vi "NEW Set Controller Limits.vi"(0 "IndMin":dbl, 1 "Min":dbl, 2 "Max":dbl, 3 "StepSize":dbl, 7 "ControlArray In":T1(array[cluster])=[{"Name"="Volt_Direct", "PI Far->Close"=[{"Slew"=1000.0, "Kp"=0.1, "Ki"=0.02}, {"Slew"=60.0, "Kp"=5.0, "Ki"=2.0}, {"Slew"=1.0, "Kp"=180.0, "Ki"=0.0}], "Limits"={"StepSize"=1e-05, "Max"=10.0, "Min"=0.0, "IndMin"=0.0}, "Cutoffs"={"Middle"=1.5, "Close"=0.2}, "FFinfo"={"FF_m"=0.5, "FF_b"=0.0}}, {"Name"="Volt_Flow", "PI Far->Close"=[{"Slew"=75.0, "Kp"=0.75, "Ki"=0.0}, {"Slew"=30.0, "Kp"=1.25, "Ki"=0.1}, {"Slew"=1.0, "Kp"=25.0, "Ki"=2.0}], "Limits"={"StepSize"=1e-05, "Max"=10.0, "Min"=0.0, "IndMin"=0.0}, "Cutoffs"={"Middle"=15.0, "Close"=4.0}, "FFinfo"={"FF_m"=0.0, "FF_b"=0.0}}, {"Name"="Volt_Speed", "PI Far->Close"=[{"Slew"=200.0, "Kp"=0.75, "Ki"=0.0}, {"Slew"=6.0, "Kp"=0.5, "Ki"=0.01}, {"Slew"=0.003, "Kp"=5.0, "Ki"=3.0}], "Limits"={"StepSize"=1e-05, "Max"=10.0, "Min"=0.0, "IndMin"=0.0}, "Cutoffs"={"Middle"=250.0, "Close"=25.0}, "FFinfo"={"FF_m"=0.0014, "FF_b"=8.5}}, {"Name"="Pres_Direct", "PI Far->Close"=[{"Slew"=25.0, "Kp"=0.4, "Ki"=0.0}, {"Slew"=2.0, "Kp"=35.0, "Ki"=0.3}, {"Slew"=0.1, "Kp"=35.0, "Ki"=0.3}], "Limits"={"StepSize"=1e-05, "Max"=5.0, "Min"=0.0, "IndMin"=0.0}, "Cutoffs"={"Middle"=30.0, "Close"=4.0}, "FFinfo"={"FF_m"=0.0, "FF_b"=0.0}}, {"Name"="Pres_Flow", "PI Far->Close"=[{"Slew"=65.0, "Kp"=-5.0, "Ki"=-10.0}, {"Slew"=25.0, "Kp"=-25.0, "Ki"=-1.0}, {"Slew"=1.0, "Kp"=-250.0, "Ki"=-120.0}], "Limits"={"StepSize"=1e-05, "Max"=5.0, "Min"=0.0, "IndMin"=0.0}, "Cutoffs"={"Middle"=15.0, "Close"=4.0}, "FFinfo"={"FF_m"=0.0, "FF_b"=0.0}}, {"Name"="Pres_Speed", "PI Far->Close"=[{"Slew"=50.0, "Kp"=-100.0, "Ki"=-10.0}, {"Slew"=1.0, "Kp"=-50.0, "Ki"=-7.5}, {"Slew"=1.0, "Kp"=-50.0, "Ki"=-7.5}], "Limits"={"StepSize"=1e-05, "Max"=5.0, "Min"=0.0, "IndMin"=0.0}, "Cutoffs"={"Middle"=250.0, "Close"=25.0}, "FFinfo"={"FF_m"=0.0, "FF_b"=0.0}}, {"Name"="CMD_Direct", "PI Far->Close"=[{"Slew"=1.0, "Kp"=1.0, "Ki"=0.1}, {"Slew"=1.0, "Kp"=1.0, "Ki"=0.1}, {"Slew"=1.0, "Kp"=1.0, "Ki"=0.1}], "Limits"={"StepSize"=0.1, "Max"=90.0, "Min"=10.0, "IndMin"=0.0}, "Cutoffs"={"Middle"=0.0, "Close"=0.0}, "FFinfo"={"FF_m"=1.0, "FF_b"=0.0}}, {"Name"="CMD_Flow", "PI Far->Close"=[{"Slew"=650.0, "Kp"=10.0, "Ki"=1.0}, {"Slew"=50.0, "Kp"=100.0, "Ki"=2.0}, {"Slew"=10.0, "Kp"=140.0, "Ki"=5.0}], "Limits"={"StepSize"=0.1, "Max"=90.0, "Min"=10.0, "IndMin"=0.0}, "Cutoffs"={"Middle"=15.0, "Close"=4.0}, "FFinfo"={"FF_m"=0.0, "FF_b"=90.0}}, {"Name"="CMD_Speed", "PI Far->Close"=[{"Slew"=999999.0, "Kp"=0.0, "Ki"=0.0}, {"Slew"=999999.0, "Kp"=0.0, "Ki"=0.0}, {"Slew"=999999.0, "Kp"=0.15, "Ki"=0.0}], "Limits"={"StepSize"=0.1, "Max"=90.0, "Min"=10.0, "IndMin"=0.0}, "Cutoffs"={"Middle"=250.0, "Close"=25.0}, "FFinfo"={"FF_m"=0.00875, "FF_b"=-2.5}}]) -> (8 "ControlArray Out":T1(array[cluster])=[{"Name"="Volt_Direct", "PI Far->Close"=[{"Slew"=1000.0, "Kp"=0.1, "Ki"=0.02}, {"Slew"=60.0, "Kp"=5.0, "Ki"=2.0}, {"Slew"=1.0, "Kp"=180.0, "Ki"=0.0}], "Limits"={"StepSize"=1e-05, "Max"=10.0, "Min"=0.0, "IndMin"=0.0}, "Cutoffs"={"Middle"=1.5, "Close"=0.2}, "FFinfo"={"FF_m"=0.5, "FF_b"=0.0}}, {"Name"="Volt_Flow", "PI Far->Close"=[{"Slew"=75.0, "Kp"=0.75, "Ki"=0.0}, {"Slew"=30.0, "Kp"=1.25, "Ki"=0.1}, {"Slew"=1.0, "Kp"=25.0, "Ki"=2.0}], "Limits"={"StepSize"=1e-05, "Max"=10.0, "Min"=0.0, "IndMin"=0.0}, "Cutoffs"={"Middle"=15.0, "Close"=4.0}, "FFinfo"={"FF_m"=0.0, "FF_b"=0.0}}, {"Name"="Volt_Speed", "PI Far->Close"=[{"Slew"=200.0, "Kp"=0.75, "Ki"=0.0}, {"Slew"=6.0, "Kp"=0.5, "Ki"=0.01}, {"Slew"=0.003, "Kp"=5.0, "Ki"=3.0}], "Limits"={"StepSize"=1e-05, "Max"=10.0, "Min"=0.0, "IndMin"=0.0}, "Cutoffs"={"Middle"=250.0, "Close"=25.0}, "FFinfo"={"FF_m"=0.0014, "FF_b"=8.5}}, {"Name"="Pres_Direct", "PI Far->Close"=[{"Slew"=25.0, "Kp"=0.4, "Ki"=0.0}, {"Slew"=2.0, "Kp"=35.0, "Ki"=0.3}, {"Slew"=0.1, "Kp"=35.0, "Ki"=0.3}], "Limits"={"StepSize"=1e-05, "Max"=5.0, "Min"=0.0, "IndMin"=0.0}, "Cutoffs"={"Middle"=30.0, "Close"=4.0}, "FFinfo"={"FF_m"=0.0, "FF_b"=0.0}}, {"Name"="Pres_Flow", "PI Far->Close"=[{"Slew"=65.0, "Kp"=-5.0, "Ki"=-10.0}, {"Slew"=25.0, "Kp"=-25.0, "Ki"=-1.0}, {"Slew"=1.0, "Kp"=-250.0, "Ki"=-120.0}], "Limits"={"StepSize"=1e-05, "Max"=5.0, "Min"=0.0, "IndMin"=0.0}, "Cutoffs"={"Middle"=15.0, "Close"=4.0}, "FFinfo"={"FF_m"=0.0, "FF_b"=0.0}}, {"Name"="Pres_Speed", "PI Far->Close"=[{"Slew"=50.0, "Kp"=-100.0, "Ki"=-10.0}, {"Slew"=1.0, "Kp"=-50.0, "Ki"=-7.5}, {"Slew"=1.0, "Kp"=-50.0, "Ki"=-7.5}], "Limits"={"StepSize"=1e-05, "Max"=5.0, "Min"=0.0, "IndMin"=0.0}, "Cutoffs"={"Middle"=250.0, "Close"=25.0}, "FFinfo"={"FF_m"=0.0, "FF_b"=0.0}}, {"Name"="CMD_Direct", "PI Far->Close"=[{"Slew"=1.0, "Kp"=1.0, "Ki"=0.1}, {"Slew"=1.0, "Kp"=1.0, "Ki"=0.1}, {"Slew"=1.0, "Kp"=1.0, "Ki"=0.1}], "Limits"={"StepSize"=0.1, "Max"=90.0, "Min"=10.0, "IndMin"=0.0}, "Cutoffs"={"Middle"=0.0, "Close"=0.0}, "FFinfo"={"FF_m"=1.0, "FF_b"=0.0}}, {"Name"="CMD_Flow", "PI Far->Close"=[{"Slew"=650.0, "Kp"=10.0, "Ki"=1.0}, {"Slew"=50.0, "Kp"=100.0, "Ki"=2.0}, {"Slew"=10.0, "Kp"=140.0, "Ki"=5.0}], "Limits"={"StepSize"=0.1, "Max"=90.0, "Min"=10.0, "IndMin"=0.0}, "Cutoffs"={"Middle"=15.0, "Close"=4.0}, "FFinfo"={"FF_m"=0.0, "FF_b"=90.0}}, {"Name"="CMD_Speed", "PI Far->Close"=[{"Slew"=999999.0, "Kp"=0.0, "Ki"=0.0}, {"Slew"=999999.0, "Kp"=0.0, "Ki"=0.0}, {"Slew"=999999.0, "Kp"=0.15, "Ki"=0.0}], "Limits"={"StepSize"=0.1, "Max"=90.0, "Min"=10.0, "IndMin"=0.0}, "Cutoffs"={"Middle"=250.0, "Close"=25.0}, "FFinfo"={"FF_m"=0.00875, "FF_b"=-2.5}}])   [LabVIEW 2013]
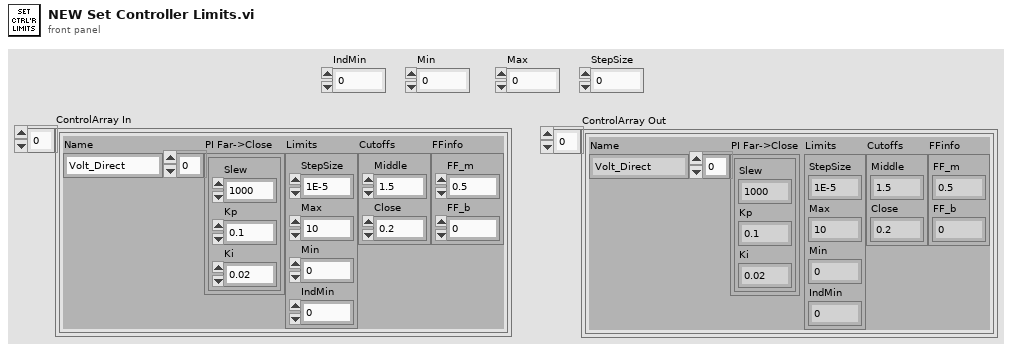
[diagram p1: front panel]
types:
  T1 = cluster{"Name":string, "PI Far->Close":cluster{"Slew":dbl, "Kp":dbl, "Ki":dbl}[], "Limits":cluster{"StepSize":dbl, "Max":dbl, "Min":dbl, "IndMin":dbl}, "Cutoffs":cluster{"Middle":dbl, "Close":dbl}, "FFinfo":cluster{"FF_m":dbl, "FF_b":dbl}}[]
  T2 = cluster{"Name":string, "PI Far->Close":cluster{"Slew":dbl, "Kp":dbl, "Ki":dbl}[], "Limits":cluster{"StepSize":dbl, "Max":dbl, "Min":dbl, "IndMin":dbl}, "Cutoffs":cluster{"Middle":dbl, "Close":dbl}, "FFinfo":cluster{"FF_m":dbl, "FF_b":dbl}}
  T3 = cluster{"StepSize":dbl, "Max":dbl, "Min":dbl, "IndMin":dbl}
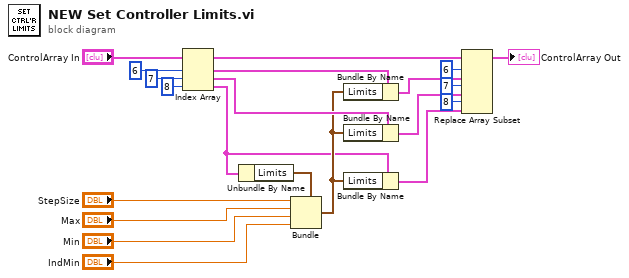
[diagram p0: block diagram]
diagram:
  n1 = Index Array(array="ControlArray In", index #1=6 ("index"), index #2=7 ("index"), index #3=8 ("index")) -> (element #1=w16:T2, element #2=w17:T2, element #3=w13:T2)
  n2 = Unbundle By Name(w13) -> ("Limits"=w15:T3)
  n3 = Bundle(cluster=w15, "StepSize"="StepSize", "Max"="Max", "Min"="Min", "IndMin"="IndMin") -> (w14:T3)
  n4 = Bundle By Name(cluster=w16, "Limits"=w14) -> (w11:T2)
  n5 = Bundle By Name(cluster=w17, "Limits"=w14) -> (w10:T2)
  n6 = Bundle By Name(cluster=w13, "Limits"=w14) -> (w9:T2)
  n7 = Replace Array Subset(array="ControlArray In", new element #1=w11, index #1=6 ("index"), new element #2=w10, index #2=7 ("index"), new element #3=w9, index #3=8 ("index")) -> (→"ControlArray Out":T1)
